vi "Do.vi"(8 "error in":errorcluster, 10 "Actor in":refnum<class "Actor.lvclass">, 11 "Clear Messages MSG":refnum<class "Clear Messages MSG.lvclass">) -> (0 "error out":errorcluster, 2 "Actor out":refnum<class "Actor.lvclass">)   [LabVIEW 2014, in "Controller.lvlib" / "Clear Messages MSG.lvclass"]
doc: "(<B>Filename</B>: Actor Framework.lvlib:Message.lvclass:Do.vi)\n\nDefines what a message does when it is received by an actor. Generally, a message instructs an actor to invoke one of its methods. By default, this method does nothing. A child class must override it to define behavior. Create a child class by using the Actor Framework Message Maker dialog box."
uses:
  Clear Messages MSG.lvclass
  <vilib>/ActorFramework/Actor/Actor.lvclass
  Controller.lvclass
  Controller.lvclass/Controller.ctl
  Accessors/Read clrMsg.vi
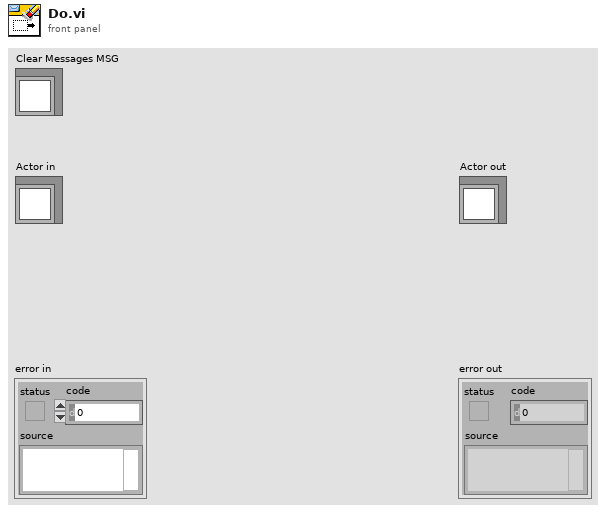
[diagram p1: front panel]
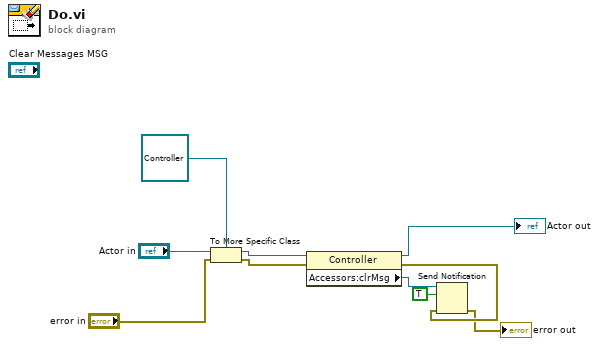
[diagram p0: block diagram]
diagram:
  n1 = To More Specific Class(target class=refnum<class "Controller.lvclass"> refnum ("Controller.lvlib:Controller"), reference="Actor in", error in="error in") -> (specific class reference=w7:refnum<class "Controller.lvclass">, error out=w6:errorcluster)
  n2 = property class="Controller"(reference=w7, error in=w6) -> (reference out=→"Actor out":refnum<class "Controller.lvclass">, error out=w3:errorcluster, "Accessors:clrMsg"=w5:refnum<notifier>)
  n3 = Send Notification(notification=TRUE, notifier=w5, error in (no error)=w3) -> (error out=→"error out":errorcluster)  [unwired: 1 out]
